vi "LS100_MES.vi"(1 "Porta COMM:":i8=1) -> (0 "L (cd/m²)":dbl)   [LabVIEW 2017]
uses:
  ls1x0cs100a.dll
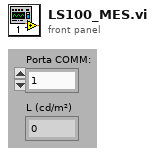
[diagram p1: front panel]
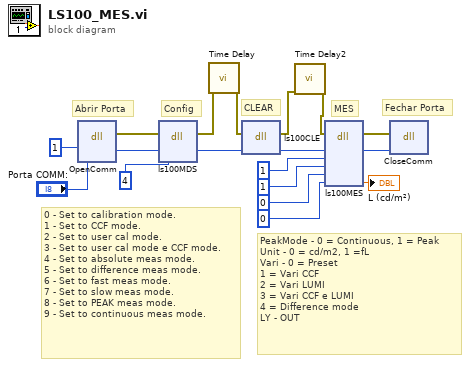
[diagram p0: block diagram]
diagram:
  # "PeakMode - 0 = Continuous, 1 = Peak\nUnit - 0 = cd/m2, 1 =fL \nVari - 0 = Preset \n1 = Vari CCF \n2 = Vari LUMI\n3 = Vari CCF e LUMI \n4 = Difference mode\nLY - OUT"
  # "0 - Set to calibration mode.\n1 - Set to CCF mode.\n2 - Set to user cal mode.\n3 - Set to user cal mode e CCF mode.\n4 - Set to absolute meas mode.\n5 - Set to difference meas mode.\n6 - Set to fast meas mode.\n7 - Set to slow meas mode.\n8 - Set to PEAK meas mode.\n9 - Set to continuous meas mode."
  # "Config"
  # "CLEAR"
  # "MES"
  # "Fechar Porta"
  # "Abrir Porta"
  n1 = dll-call lib="C:/LabViewDrivers/LS100/ls1x0cs100a.dll" fn="OpenComm"("fNum"=i8 1, "PortNumber"="Porta COMM:") -> (error out=w1:errorcluster, "fNum"=w9:i8)  [unwired: 5 in, 1 out]
  n2 = dll-call lib="C:/LabViewDrivers/LS100/ls1x0cs100a.dll" fn="ls100MDS"(error in=w1, "fNum"=w9, "Mode"=i8 4) -> (error out=w6:errorcluster, "fNum"=w17:i8)  [unwired: 4 in, 1 out]
  n3 = call "Time Delay"("error in (no error)"=w6) -> ("error out"=w5:errorcluster)  [unwired: 10 in]
  n4 = dll-call lib="C:/LabViewDrivers/LS100/ls1x0cs100a.dll" fn="ls100CLE"(error in=w5, "fnum"=w17) -> (error out=w4:errorcluster, "fnum"=w16:i8)  [unwired: 3 in, 1 out]
  n5 = call "Time Delay2"("error in (no error)"=w4) -> ("error out"=w3:errorcluster)  [unwired: 10 in]
  n6 = dll-call lib="C:/LabViewDrivers/LS100/ls1x0cs100a.dll" fn="ls100MES"(error in=w3, "fNum"=w16, "PeakMode"=i8 1, "Unit"=i8 1, "Vari"=i8 0, "LY"=i16 0) -> (error out=w2:errorcluster, "fNum"=w8:i8, "LY"=→"L (cd/m²)":dbl)  [unwired: 6 in, 1 out]
  n7 = dll-call lib="C:/LabViewDrivers/LS100/ls1x0cs100a.dll" fn="CloseComm"(error in=w2, "fNum"=w8) -> ()  [unwired: 4 in, 2 out]
